vi "adam-5000-set-DO.vi"(6 "send command":bool, 7 "ack in":string, 8 "error in (no error)":errorcluster, 9 "Output State":bool, 10 "DO Number":u8, 11 "VISA Refnum in":refnum<visa-resource-name>) -> (0 "error out":errorcluster, 1 "success?":bool, 2 "read buffer out":string, 3 "VISA Refnum out":refnum<visa-resource-name>, 4 "Command Used":string, 5 "acknowledge char":string)   [LabVIEW 2020]
uses:
  <vilib>/Instr/_visa.llb/VISA Configure Serial Port (Instr).vi
panel:
  in  "Chassis Slot":u8=3
  out "read return":u32
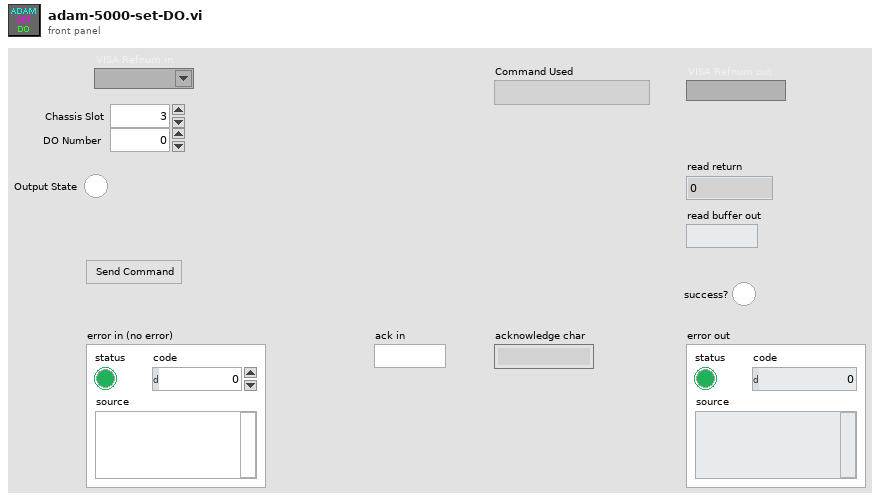
[diagram p1: front panel]
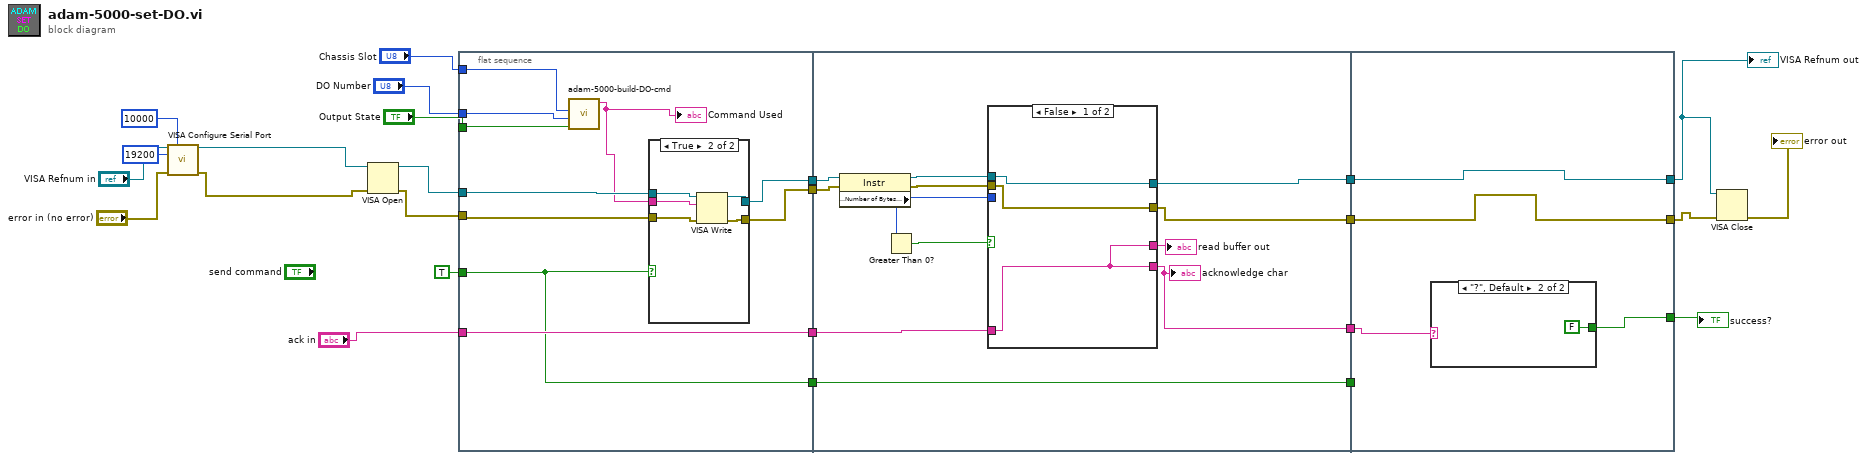
[diagram p0: block diagram]
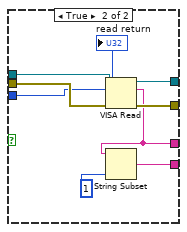
[diagram p3: hidden frame]
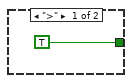
[diagram p4: hidden frame]
diagram:
  n1 = call-poly "VISA Configure Serial Port"("VISA resource name"="VISA Refnum in", "timeout (10sec)"=u32 10000, "baud rate (9600)"=u32 19200, "error in (no error)"="error in (no error)") -> ("VISA resource name out"=w6:refnum<visa-resource-name>, "error out"=w2:errorcluster)  [unwired: 10 in]
  n2 = VISA Open(error in (no error)=w2, VISA resource name=w6) -> (VISA resource name=w12:refnum<visa-resource-name>, error out=w11:errorcluster)  [unwired: 3 in]
  n3 = flat-sequence {
    tunnel: "ack in" -> [w35]
    tunnel: TRUE ("send command") -> [w34]
    tunnel: [w34] -> w21
    tunnel: [w35] -> w20
    tunnel: [w31] -> w19
    tunnel: [w30] -> w18
    tunnel: w12 -> [w33]
    tunnel: w11 -> [w32]
    tunnel: "Output State" -> [w29]
    tunnel: "DO Number" -> [w28]
    tunnel: "Chassis Slot" -> [w26]
    tunnel: [w45] -> w24
    tunnel: [w54] -> w23
    tunnel: w21 -> [w54]
    tunnel: w20 -> [w48]
    tunnel: w19 -> [w47]
    tunnel: w18 -> [w46]
    tunnel: [w44] -> w15
    tunnel: [w43] -> w14
    tunnel: [w69] -> w25
    tunnel: w24 -> [w70]
    tunnel: w23 -> [_]
    tunnel: [w68] -> w10
    tunnel: w15 -> [w68]
    tunnel: w14 -> [w67]
    tunnel: [w67] -> w9
    frame #0 {
      n4 = call "adam-5000-build-DO-cmd.vi"("Output State"=w29, "DO Number"=w28, "Chassis Slot"=w26) -> ("Command Out"=w27:string)  [unwired: 8 in]
      "Command Used" <- w27
      n5 = case shown="True" w34 {
        tunnel: w33 -> [w37 w42]
        tunnel: w32 -> [w36 w41]
        tunnel: w27 -> [_ w40]
        tunnel: [w37 w39] -> w31
        tunnel: [w36 w38] -> w30
        frame False {
        }
        frame True {
          n6 = VISA Write(VISA resource name=w42, write buffer=w40, error in (no error)=w41) -> (VISA resource name out=w39:refnum<visa-resource-name>, error out=w38:errorcluster)  [unwired: 1 out]
        }
      }
    }
    frame #1 {
      n7 = property class="Instr"(reference=w47, error in=w46) -> (reference out=w51:refnum<visa-resource-name>, error out=w52:errorcluster, "Serial Settings:Number of Bytes at Serial Port"=w50:u32)
      n8 = Greater Than 0?(x=w50) -> (x > 0?=w49:bool)
      n9 = case shown="False" w49 {
        tunnel: w52 -> [w57 w66]
        tunnel: w51 -> [w56 w65]
        tunnel: [w55 w63] -> w45
        tunnel: [w57 w62] -> w43
        tunnel: [w56 w60] -> w44
        tunnel: w50 -> [_ w59]
        tunnel: w48 -> [w55 _]
        tunnel: [w55 w58] -> w53
        frame False {
        }
        frame True {
          n10 = VISA Read(VISA resource name=w65, byte count=w59, error in (no error)=w66) -> (VISA resource name out=w60:refnum<visa-resource-name>, read buffer=w58:string, return count=→"read return":u32, error out=w62:errorcluster)
          n11 = String Subset(string=w58, length (rest)=1 ("length (rest)")) -> (substring=w63:string)  [unwired: 1 in]
        }
      }
      "acknowledge char" <- w45
      "read buffer out" <- w53
    }
    frame #2 {
      n12 = case shown="\"?\", Default" w70 {
        tunnel: [TRUE ("success?") FALSE ("success?")] -> w69
        frame ">" {
        }
        frame "?", Default {
        }
      }
    }
  }
  n13 = VISA Close(VISA resource name=w10, error in (no error)=w9) -> (error out=→"error out":errorcluster)
  "success?" <- w25
  "VISA Refnum out" <- w10
